vi "Set DG535 for FPGA.vi"(8 "error in (no error)":errorcluster, 11 "GPIB address":string) -> (0 "error out":errorcluster)   [LabVIEW 2013]
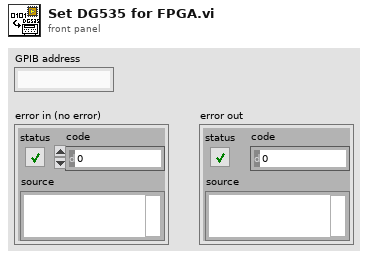
[diagram p1: front panel]
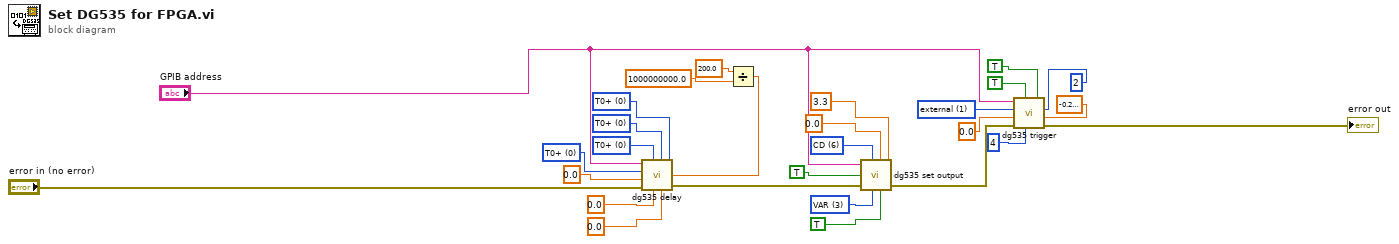
[diagram p0: block diagram]
diagram:
  w12 = u32 1 items=["internal", "external", "single shot", "burst", "line"] ("trigger")
  w10 = 3 items=["TTL", "NIM", "ECL", "VAR"] ("mode")
  w8 = u16 6 items=["T0", "A", "B", "AB", "C", "D", "CD"] ("output")
  w5 = u32 0 items=["T0+", "A+", "B+", "C+"] ("D=")
  w4 = u32 0 items=["T0+", "A+", "B+", "D+"] ("C=")
  w3 = u32 0 items=["T0+", "A+", "C+", "D+"] ("B=")
  w2 = u32 0 items=["T0+", "B+", "C+", "D+"] ("A=")
  n1 = Divide(x=200.0 ("D"), y=1000000000.0) -> (x/y=w26:dbl)
  n2 = call "dg535 delay.vi"("C"=0.0, "D"=w26, "D="=w5, "C="=w4, "B"=0.0 ("C"), "error in"="error in (no error)", "A"=0.0 ("D"), "B="=w3, "A="=w2, "GPIB address"="GPIB address") -> ("error out"=w6:errorcluster)
  n3 = call "dg535 set output.vi"("GPIB address"="GPIB address", "output"=w8, "set"=TRUE, "error in"=w6, "mode"=w10, "offset"=0.0, "amplitude"=3.3, "load"=TRUE) -> ("error out"=w19:errorcluster)  [unwired: 1 in]
  n4 = call "dg535 trigger.vi"("external trigger level"=sgl -0.2, "burst count"=2, "trigger slope"=TRUE, "burst period"=4, "input impedance"=TRUE, "error in"=w19, "internal/burst trigger rate"=0.0, "trigger"=w12, "GPIB address"="GPIB address") -> ("error out"=→"error out":errorcluster)
